vi "Camera Global Data.vi"() -> ()   [LabVIEW 2013]
panel:
  in  "Camera Global Data":T1
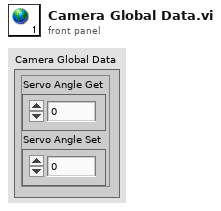
[diagram p1: front panel]
types:
  T1 = cluster{"Servo Angle Get":dbl, "Servo Angle Set":dbl}
diagram:
